vi "Main Page.vi"(8 "error in (no error)":errorcluster, 11 "Node Ptr":T3 format="%.0x") -> (0 "error out":errorcluster)   [LabVIEW 2018, in "Instrument Addon System Explorer.lvlib"]
uses:
  Instrument Addon System Explorer.lvlib
  <vilib>/NI Veristand/Custom Device API/Custom Device Item Ref.ctl
  Addon Shared/Types/FG Control.ctl
  <vilib>/NI/NI VeriStand Hardware Resource Discovery/_Types/Filter Type.ctl
  Addon Shared/SubVIs/Constants.vi
  <vilib>/NI/NI VeriStand Advanced SysDef API/SysDef API/SysDef.Property.Get.vi
  <vilib>/NI/NI VeriStand Advanced SysDef API/_SubVIs/SysDef.Property.Get.String.vi
  <vilib>/NI/NI VeriStand Advanced SysDef API/SysDef API/SysDef.Property.Set.vi
  <vilib>/NI/NI VeriStand Advanced SysDef API/_SubVIs/SysDef.Property.Set.String.vi
  <vilib>/NI Veristand/Custom Device API/NI VeriStand - Get Item Property.vi
  <vilib>/NI Veristand/Custom Device API/Get Item Property (Boolean).vi
  <vilib>/NI Veristand/Custom Device API/Get Item Property (U32).vi
  <vilib>/NI Veristand/Custom Device API/Get Item Property (String).vi
  <vilib>/NI Veristand/Custom Device API/NI VeriStand - Set Item Property.vi
  <vilib>/NI Veristand/Custom Device API/Set Item Property (Boolean).vi
  <vilib>/NI Veristand/Custom Device API/Set Item Property (U32).vi
  <vilib>/NI Veristand/Custom Device API/Set Item Property (String).vi
  <vilib>/Utility/LVClass/Get LV Class Default Value.vi
  Support Libraries/Protocols.lvlibp/Protocol Parent/Protocol Parent.lvclass
  <vilib>/NI Veristand/Custom Device API/Custom Device API.lvlib
  Addon Shared/Instrument Addon Shared.lvlib
  <vilib>/NI/NI VeriStand Hardware Resource Discovery/NIVS Hardware Discovery.lvlib
  APIs/Scripting API/Instrument Addon Scripting API.lvlib
panel:
  out "Version":string
  in  "PCL Decimation":u32=1 min=1 max=10000 step=1
  in  "Protocol Settings":T1(tab)=enum."TCP/IP"
  in  "COM Browse":bool
  in  "Termination Character":u8=10 format="%.0x"
  in  "End Write":bool=TRUE caption="End Write on Termination Character?"
  in  "End Read":bool=TRUE caption="End Read on Termination Character?"
  in  "XOFF":T2(ring)=enum."DC3"
  in  "XON":T2(ring)=enum."DC1"
  in  "Flow Control":u16(ring) items=["None"=0, "XON/XOFF"=1, "RTS/CTS"=2, "DTR/DSR"=4]
  in  "Stop Bits":u16(ring)=10 items=["1.0"=10, "1.5"=15, "2.0"=20]
  in  "Parity":enum16{"None", "Odd", "Even", "Mark", "Space"}(ring)
  in  "Data Bits":u16=8 min=5 max=8 step=1
  in  "Baud Rate":u32(ring)=9600 items=["75"=75, "110"=110, "134"=134, "150"=150, "300"=300, "600"=600, "1200"=1200, "1800"=1800, "2400"=2400, "4800"=4800, "7200"=7200, "9600"=9600, "14400"=14400, "19200"=19200, "28800"=28800, "38400"=38400, "56000"=56000, "57600"=57600, "115200"=115200, "128000"=128000, "230400"=230400, "460800"=460800, "921600"=921600, "1843200"=1843200, "3000000"=3000000]
  in  "Port":string="COM1"
  in  "VISA Browse":bool
  in  "Append Write Termination Character":bool caption="Append Write Termination Character?"
  in  "Timeout":u32=2000 caption="Timeout (ms)"
  in  "Termination Character":u8=10 format="%.0x"
  in  "Enable Termination Character":bool=TRUE caption="Enable Termination Character?"
  in  "VISA Resource":string="GPIB0::2::INSTR"
  in  "Port":u16
  in  "IP Address":string="localhost"
  in  "UDP Browse":bool
  in  "Target Port":u16
  in  "Target IP Address":string="localhost"
  in  "Local Port":u16
  in  "Local IP Address":string="localhost"
  in  "Assert REN w/ IFC":bool=TRUE caption="Assert REN w/ IFC?"
  in  "IST Bit Sense":bool=TRUE caption="IST Bit Sense?"
  in  "System Controller":bool=TRUE caption="System Controller?"
  in  "GPIB Address":string="1"
  in  "ConvBox Address":string="0"
  in  "ConvBox Browse":bool
  in  "ConvBox Port":string="COM1"
  in  "Protocol":string(combo)
  in  "SHDocVw.IWebBrowser":refnum<k7>(container)
  in  "Header":cluster{"Section Name":string}={"Section Name"="Addon Settings"}
  in  "Description":string
  in  "Name":string
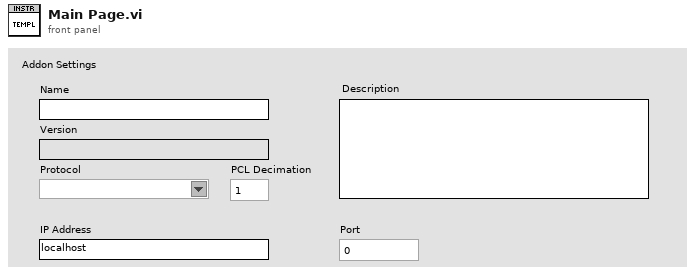
[diagram p1: front panel]
types:
  T1 = enum32{"RS232", "VISA", "TCP/IP", "UDP", "ConvBox"}
  T2 = enum16{"NUL", "SOH", "STX", "ETX", "EOT", "ENQ", "ACK", "BEL", "BS", "HT", "LF", "VT", "FF", "CR", "SO", "SI", "DLE", "DC1", "DC2", "DC3", "DC4", "NAK", "SYN", "ETB", "CAN", "EM", "SUB", "ESC", "FS", "GS", "RS", "US", "SP", "!", "\"", "#", "$", "%", "&", "'", "(", ")", "*", "+", ",", "- (-)", ".", "/", "0", "1", "2", "3", "4", "5", "6", "7", "8", "9", ":", ";", "<", "=", ">", "?", "@", "A", "B", "C", "D", "E", "F", "G", "H", "I", "J", "K", "L", "M", "N", "O", "P", "Q", "R", "S", "T", "U", "V", "W", "X", "Y", "Z", "[", "\\", "]", "^", "_", "`", "a", "b", "c", "d", "e", "f", "g", "h", "i", "j", "k", "l", "m", "n", "o", "p", "q", "r", "s", "t", "u", "v", "w", "x", "y", "z", "{", "|", "}", "~"}
  T3 = typedef "Custom Device API.lvlib/Custom Device Item Ref.ctl" = u64
  T4 = typedef "Custom Device API.lvlib/Custom Device Item Info.ctl" = cluster{"Name":string, "Is Channel":bool, "GUID":string, "Is Waveform":bool}
  T5 = typedef "Instrument Addon Shared.lvlib/FG Control.ctl" = enum16{"Get", "Set"}
  T6 = typedef "NIVS Hardware Discovery.lvlib/Filter Type.ctl" = enum16{"Device Category", "Product Name", "Ethernet", "XNET", "VISA", "FPGA", "EtherCAT Master", "DAQmx", "GPIB", "Serial"}
  T7 = typedef "Custom Device API.lvlib/Custom Device Commands.ctl" = enum16{"Default", "Item renamed", "Shutdown", "Dynamic button pressed"}
  T8 = typedef "Instrument Addon Shared.lvlib/VISA Settings.ctl" = cluster{"VISA Resource":string, "Enable Termination Character":bool, "Termination Character":u8, "Timeout":u32, "Append Write Termination Character":bool}
  T9 = typedef "Instrument Addon Shared.lvlib/TCPIP Settings.ctl" = cluster{"IP Address":string, "Port":u16}
  T10 = typedef "Instrument Addon Shared.lvlib/UDP Settings.ctl" = cluster{"Local IP Address":string, "Local Port":u16, "Target IP Address":string, "Target Port":u16}
  T11 = typedef "Instrument Addon Shared.lvlib/RSXXX Port Settings.ctl" = cluster{"Port":string, "Baud Rate":u32, "Data Bits":u16, "Parity":enum16{"None", "Odd", "Even", "Mark", "Space"}, "Stop Bits":u16, "Flow Control":u16, "XON":enum16{"NUL", "SOH", "STX", "ETX", "EOT", "ENQ", "ACK", "BEL", "BS", "HT", "LF", "VT", "FF", "CR", "SO", "SI", "DLE", "DC1", "DC2", "DC3", "DC4", "NAK", "SYN", "ETB", "CAN", "EM", "SUB", "ESC", "FS", "GS", "RS", "US", "SP", "!", "\"", "#", "$", "%", "&", "'", "(", ")", "*", "+", ",", "- (-)", ".", "/", "0", "1", "2", "3", "4", "5", "6", "7", "8", "9", ":", ";", "<", "=", ">", "?", "@", "A", "B", "C", "D", "E", "F", "G", "H", "I", "J", "K", "L", "M", "N", "O", "P", "Q", "R", "S", "T", "U", "V", "W", "X", "Y", "Z", "[", "\\", "]", "^", "_", "`", "a", "b", "c", "d", "e", "f", "g", "h", "i", "j", "k", "l", "m", "n", "o", "p", "q", "r", "s", "t", "u", "v", "w", "x", "y", "z", "{", "|", "}", "~"}, "XOFF":enum16{"NUL", "SOH", "STX", "ETX", "EOT", "ENQ", "ACK", "BEL", "BS", "HT", "LF", "VT", "FF", "CR", "SO", "SI", "DLE", "DC1", "DC2", "DC3", "DC4", "NAK", "SYN", "ETB", "CAN", "EM", "SUB", "ESC", "FS", "GS", "RS", "US", "SP", "!", "\"", "#", "$", "%", "&", "'", "(", ")", "*", "+", ",", "- (-)", ".", "/", "0", "1", "2", "3", "4", "5", "6", "7", "8", "9", ":", ";", "<", "=", ">", "?", "@", "A", "B", "C", "D", "E", "F", "G", "H", "I", "J", "K", "L", "M", "N", "O", "P", "Q", "R", "S", "T", "U", "V", "W", "X", "Y", "Z", "[", "\\", "]", "^", "_", "`", "a", "b", "c", "d", "e", "f", "g", "h", "i", "j", "k", "l", "m", "n", "o", "p", "q", "r", "s", "t", "u", "v", "w", "x", "y", "z", "{", "|", "}", "~"}, "End Read on Termination Character":bool, "End Write on Termination Character":bool, "Termination Character":u8}
  T12 = typedef "Instrument Addon Shared.lvlib/GPIB ConvBox Settings.ctl" = cluster{"Port":string, "ConvBox Address":string, "Assert Ren with IFC":bool, "System controller":bool, "IST bit sense":bool, "GPIB Address":string}
  T13 = typedef "Protocols.lvlibp/Protocol Parent.lvclass/Base Protocol Type.ctl" = enum16{"RS-XXX", "VISA", "TCPIP", "UDP", "GPIB ConvBox"}
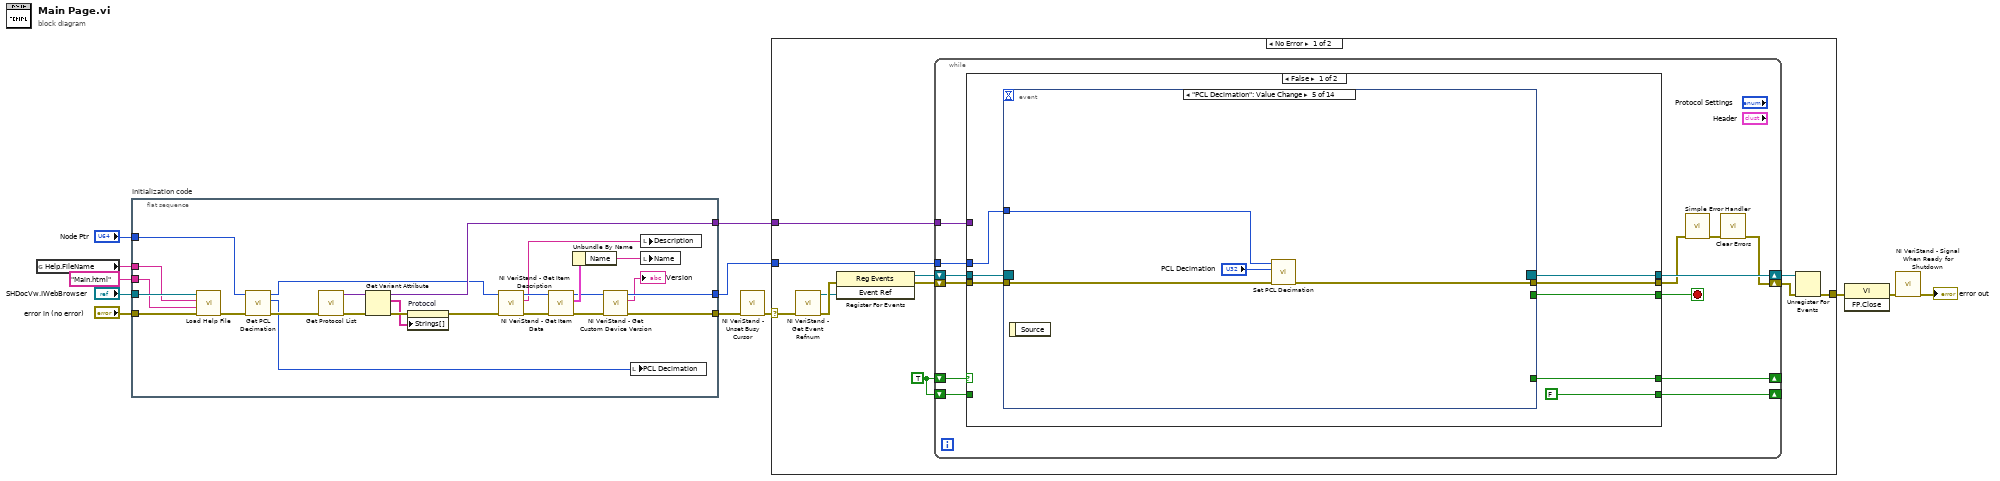
[diagram p0: block diagram]
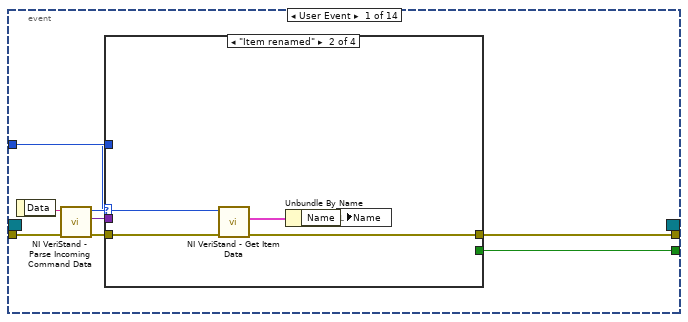
[diagram p2: hidden frame]
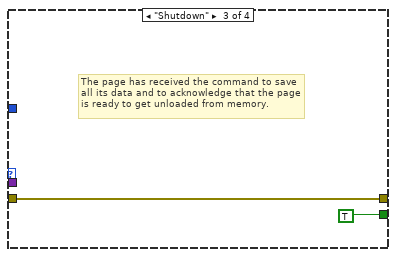
[diagram p4: hidden frame]
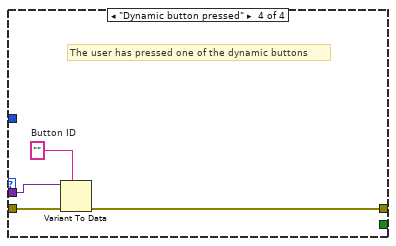
[diagram p5: hidden frame]
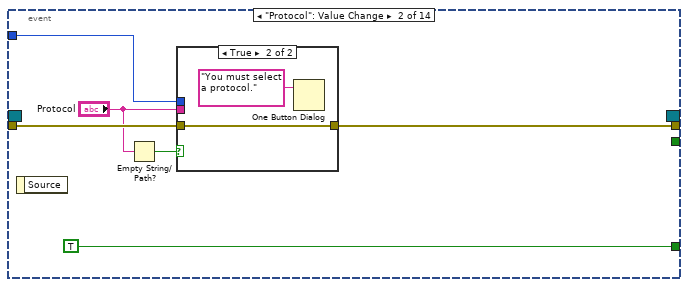
[diagram p6: hidden frame]
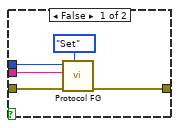
[diagram p7: hidden frame]
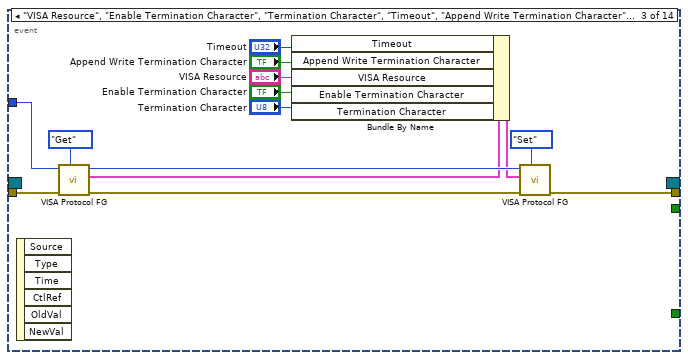
[diagram p8: hidden frame]
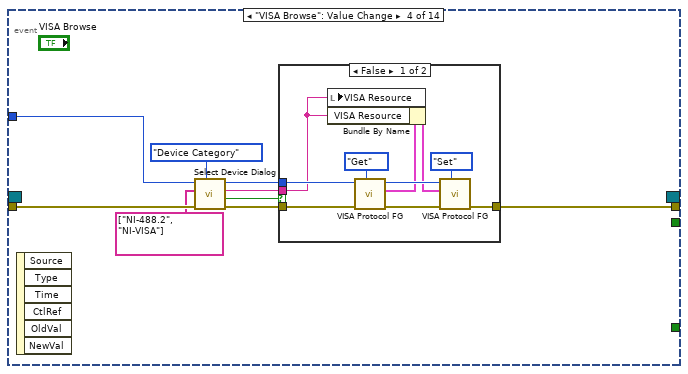
[diagram p9: hidden frame]
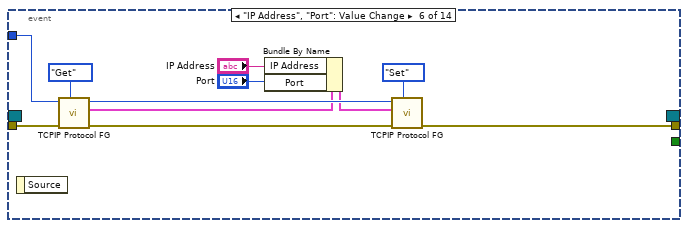
[diagram p11: hidden frame]
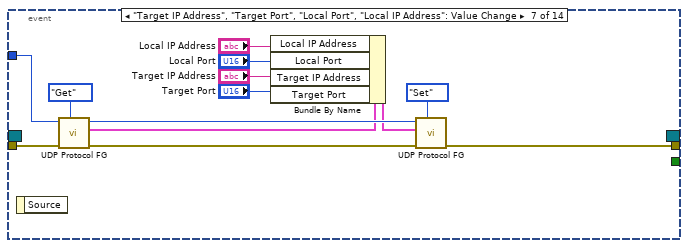
[diagram p12: hidden frame]
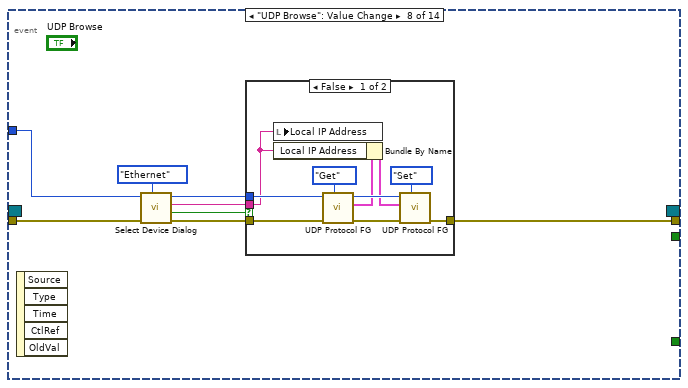
[diagram p13: hidden frame]
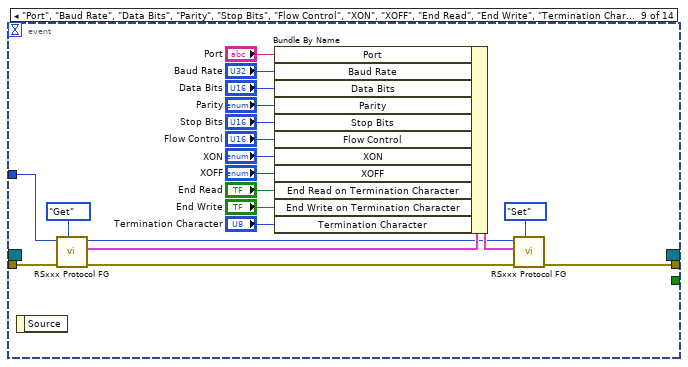
[diagram p15: hidden frame]
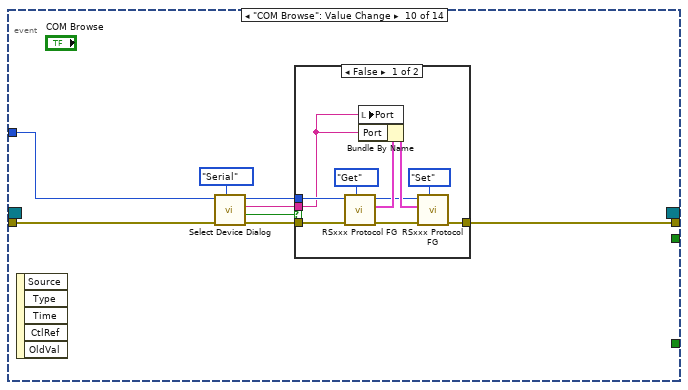
[diagram p16: hidden frame]
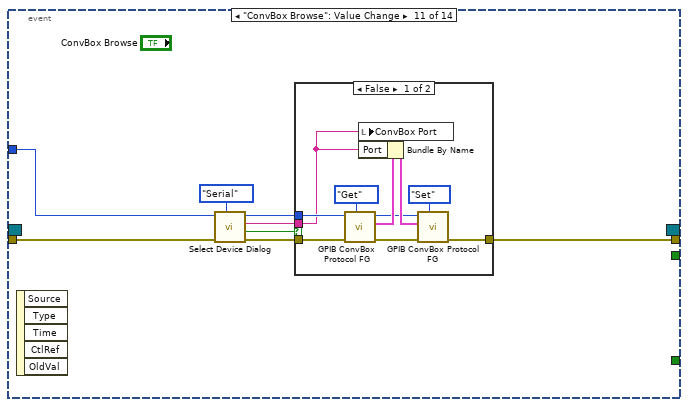
[diagram p18: hidden frame]
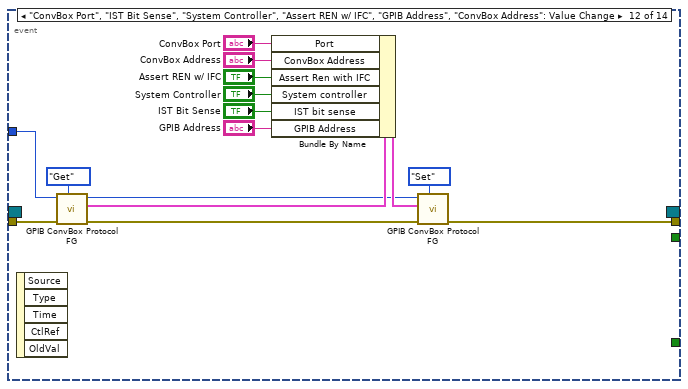
[diagram p20: hidden frame]
diagram:
  n1 = global read "Constants.vi" "Help.FileName"() -> (w1:string)
  n2 = flat-sequence "Initialization code" {
    tunnel: "error in (no error)" -> [w32]
    tunnel: "Node Ptr" -> [w16]
    tunnel: [w21] -> w8
    tunnel: [w19] -> w5
    tunnel: "SHDocVw.IWebBrowser" -> [w31]
    tunnel: "Main.html" ("HTML File") -> [w30]
    tunnel: w1 -> [w29]
    tunnel: [w24] -> w2
    frame #0 {
      n3 = call "Load Help File.vi"("error in (no error)"=w32, "HTML File"=w30, "Main CHM File"=w29, "SHDocVw.IWebBrowser2"=w31) -> ("error out"=w15:errorcluster)  [unwired: 7 in]
      n4 = call "Get PCL Decimation.vi"("Error In"=w15, "Instrument Addon Refnum In"=w16) -> ("Error Out"=w14:errorcluster, "PCL Decimation"=w13:u32, "Instrument Addon Refnum Out"=w17:T3)  [unwired: 7 in]
      n5 = call "Get Protocol List.vi"("error in (no error)"=w14) -> ("error out"=w27:errorcluster, "Class Lookup"=w28:variant)  [unwired: 9 in]
      n6 = Get Variant Attribute(Variant=w28, error in=w27) -> (duplicate Variant=w24:variant, names=w25:string[], error out=w26:errorcluster)  [unwired: 2 in, 1 out]
      n7 = property on="Protocol" class="CmbBox"(error in=w26, "Strings[]"=w25) -> (error out=w23:errorcluster)  [unwired: 1 in, 1 out]
      n8 = call <vilib>:"NI VeriStand - Get Item Description.vi"("error in (no error)"=w23, "Item Ref in"=w17) -> ("error out"=w35:errorcluster, "Description"=w36:string, "Item Ref out"=w37:T3)  [unwired: 7 out]
      n9 = call <vilib>:"NI VeriStand - Get Item Data.vi"("error in (no error)"=w35, "Item Ref in"=w37) -> ("error out"=w22:errorcluster, "Item Info"=w34:T4, "Item Ref out"=w20:T3)  [unwired: 7 out]
      n10 = Unbundle By Name(w34) -> ("Name"=w33:string)
      n11 = call <vilib>:"NI VeriStand - Get Custom Device Version.vi"("error in (no error)"=w22, "Device Ref in"=w20) -> ("error out"=w21:errorcluster, "Value"=→"Version":string, "Device Ref out"=w19:T3)  [unwired: 7 in]
      n12 = local write "PCL Decimation"(w13) -> ()
      n13 = local write "Description"(w36) -> ()
      n14 = local write "Name"(w33) -> ()
    }
  }
  n15 = call <vilib>:"NI VeriStand - Unset Busy Cursor.vi"("error in (no error)"=w8) -> ("error out"=w7:errorcluster)  [unwired: 10 out]
  n16 = case shown="No Error" w7 {
    selector: w7 -> [w40 w347]
    tunnel: [w45 w345] -> w12
    tunnel: w5 -> [w41 _]
    tunnel: w2 -> [w39 _]
    frame No Error {
      w38 = TRUE
      n17 = call <vilib>:"NI VeriStand - Get Event Refnum.vi"("error in (no error)"=w40) -> ("error out"=w48:errorcluster, "Event Ref"=w44:refnum<user-event>)  [unwired: 9 out]
      n18 = register-events(error in=w48, w44) -> (reference out=w42:refnum<event-registration>, error out=w43:errorcluster)  [unwired: 1 in]
      n19 = while {
        tunnel: w41 -> [w57]
        shift-right: [w54] -> w46
        shift-left: w43 -> [w60]
        shift-right: [w61] -> w47
        shift-left: w42 -> [w59]
        tunnel: w39 -> [w53]
        shift-right: [w51] -> _
        shift-left: w38 -> [w52]
        shift-right: [w49] -> _
        shift-left: w38 -> [w50]
        stop <- w58 stop-if-true
        n20 = case shown="False" w52 {
          tunnel: [w69 w272] -> w61
          tunnel: w60 -> [w68 w280]
          tunnel: w59 -> [w67 w272]
          tunnel: [w66 _] -> w58
          tunnel: w57 -> [w65 w279]
          tunnel: [w64 w267] -> w56
          tunnel: w53 -> [_ w277]
          tunnel: [w63 w265] -> w51
          tunnel: w50 -> [_ w266]
          tunnel: [FALSE w265] -> w49
          frame False {
            n21 = event shown="[4] \"PCL Decimation\": Value Change" {
              selector: w67 -> [_ _ _ _ _ _ _ _ _ _ _ _ _ _]
              dyn-events: [_ _ _ _ _ _ _ _ _ _ _ _ _ _] -> w69
              timeout: _ -> [_ _ _ _ _ _ _ _ _ _ _ _ _ _]
              tunnel: w68 -> [w77 w94 w115 w124 w139 w150 w163 w171 w200 w210 w229 w249 w260 w263]
              tunnel: [w73 _ _ _ _ _ _ _ _ _ _ _ _ _] -> w66
              tunnel: [w72 w90 w111 w125 w138 w146 w159 w172 w202 w211 w230 w256 w259 w262] -> w64
              tunnel: w65 -> [w71 w95 w114 w122 w137 w149 w162 w169 w198 w209 w228 w248 w258 w264]
              tunnel: [_ TRUE _ _ _ _ _ _ _ _ _ _ _ _] -> w63
              event User Event {
                n22 = event-data() -> ("Data"=w76:string)  [unwired: 1 out]
                n23 = call <vilib>:"NI VeriStand - Parse Incoming Command Data.vi"("error in (no error)"=w77, "Incoming data"=w76) -> ("error out"=w75:errorcluster, "Outgoing data"=w70:variant, "Action"=w74:T7)  [unwired: 7 out]
                n24 = case shown="\"Item renamed\"" w74 {
                  tunnel: w75 -> [w78 w83 w84 w89]
                  tunnel: [_ _ TRUE _] -> w73
                  tunnel: [w78 w80 w84 w86] -> w72
                  tunnel: w71 -> [_ w82 _ _]
                  tunnel: w70 -> [_ _ _ w88]
                  frame "Default", Default {
                  }
                  frame "Item renamed" {
                    n25 = call <vilib>:"NI VeriStand - Get Item Data.vi"("error in (no error)"=w83, "Item Ref in"=w82) -> ("error out"=w80:errorcluster, "Item Info"=w81:T4)  [unwired: 8 out]
                    n26 = Unbundle By Name(w81) -> ("Name"=w79:string)
                    n27 = local write "Name"(w79) -> ()
                  }
                  frame "Shutdown" {
                    # "The page has received the command to save all its data and to acknowledge that the page is ready to get unloaded from memory."
                  }
                  frame "Dynamic button pressed" {
                    w87 = ""  # Button ID
                    # "The user has pressed one of the dynamic buttons"
                    n28 = Variant To Data(error in=w89, type=w87, Variant=w88) -> (error out=w86:errorcluster)  [unwired: 1 out]
                  }
                }
              }
              event "Protocol": Value Change {
                n29 = event-data() -> ()  [unwired: 2 out]
                n30 = Empty String/Path?(string/path="Protocol") -> (empty?=w92:bool)
                n31 = case shown="True" w92 {
                  tunnel: w95 -> [w98 _]
                  tunnel: w94 -> [w99 w101]
                  tunnel: [w96 w101] -> w90
                  tunnel: "Protocol" -> [w97 _]
                  frame False {
                    n32 = call "Protocol FG.vi"("Action"=FG_Control."Set", "error in (no error)"=w99, "Protocol"=w97, "Device Item Ref in"=w98) -> ("error out"=w96:errorcluster)  [unwired: 5 in, 2 out]
                  }
                  frame True {
                    n33 = One Button Dialog(message="You must select a protocol.") -> ()  [unwired: 1 in, 1 out]
                  }
                }
              }
              event "VISA Resource", "Enable Termination Character", "Termination Character", "Timeout", "Append Write Termination Character": Value Change {
                n34 = event-data() -> ()  [unwired: 7 out]
                n35 = call "VISA Protocol FG.vi"("Action"=FG_Control."Get", "error in (no error)"=w115, "Device Item Ref in"=w114) -> ("error out"=w112:errorcluster, "VISA Config"=w109:T8, "Item Ref out"=w110:T3)  [unwired: 6 in]
                n36 = Bundle By Name(cluster=w109, "Timeout"="Timeout", "Append Write Termination Character"="Append Write Termination Character", "VISA Resource"="VISA Resource", "Enable Termination Character"="Enable Termination Character", "Termination Character"="Termination Character") -> (w108:T8)
                n37 = call "VISA Protocol FG.vi"("Action"=FG_Control."Set", "error in (no error)"=w112, "VISA Config"=w108, "Device Item Ref in"=w110) -> ("error out"=w111:errorcluster)  [unwired: 5 in, 2 out]
              }
              event "VISA Browse": Value Change {
                n38 = event-data() -> ()  [unwired: 7 out]
                n39 = call <vilib>:"Select Device Dialog.vi"("Filter Type"=Filter_Type."Device Category", "error in (no error)"=w124, "Filter Names"=string[] ["NI-488.2", "NI-VISA"], "Item Ref in"=w122) -> ("error out"=w123:errorcluster, "Cancelled?"=w120:bool, "Selected Alias"=w119:string, "Item Ref out"=w121:T3)  [unwired: 4 in]
                n40 = case shown="False" w120 {
                  tunnel: w123 -> [w134 w136]
                  tunnel: w121 -> [w133 _]
                  tunnel: [w130 w136] -> w125
                  tunnel: w119 -> [w126 _]
                  frame False {
                    n41 = local write "VISA Resource"(w126) -> ()
                    n42 = call "VISA Protocol FG.vi"("Action"=FG_Control."Get", "error in (no error)"=w134, "Device Item Ref in"=w133) -> ("error out"=w131:errorcluster, "VISA Config"=w128:T8, "Item Ref out"=w129:T3)  [unwired: 6 in]
                    n43 = Bundle By Name(cluster=w128, "VISA Resource"=w126) -> (w127:T8)
                    n44 = call "VISA Protocol FG.vi"("Action"=FG_Control."Set", "error in (no error)"=w131, "VISA Config"=w127, "Device Item Ref in"=w129) -> ("error out"=w130:errorcluster)  [unwired: 5 in, 2 out]
                  }
                  frame True {
                  }
                }
              }
              event "PCL Decimation": Value Change {
                n45 = event-data() -> ()  [unwired: 2 out]
                n46 = call "Set PCL Decimation.vi"("Error In"=w139, "PCL Decimation"="PCL Decimation", "Instrument Addon Refnum In"=w137) -> ("Error Out"=w138:errorcluster)  [unwired: 7 in, 1 out]
              }
              event "IP Address", "Port": Value Change {
                n47 = event-data() -> ()  [unwired: 2 out]
                n48 = call "TCPIP Protocol FG.vi"("Action"=FG_Control."Get", "error in (no error)"=w150, "Device Item Ref in"=w149) -> ("error out"=w147:errorcluster, "TCP/IP Config"=w144:T9, "Item Ref out"=w145:T3)  [unwired: 6 in]
                n49 = Bundle By Name(cluster=w144, "IP Address"="IP Address", "Port"="Port") -> (w143:T9)
                n50 = call "TCPIP Protocol FG.vi"("Action"=FG_Control."Set", "error in (no error)"=w147, "TCP/IP Config"=w143, "Device Item Ref in"=w145) -> ("error out"=w146:errorcluster)  [unwired: 5 in, 2 out]
              }
              event "Target IP Address", "Target Port", "Local Port", "Local IP Address": Value Change {
                n51 = event-data() -> ()  [unwired: 2 out]
                n52 = call "UDP Protocol FG.vi"("Action"=FG_Control."Get", "error in (no error)"=w163, "Device Item Ref in"=w162) -> ("error out"=w160:errorcluster, "UDP Config"=w157:T10, "Item Ref out"=w158:T3)  [unwired: 6 in]
                n53 = Bundle By Name(cluster=w157, "Local IP Address"="Local IP Address", "Local Port"="Local Port", "Target IP Address"="Target IP Address", "Target Port"="Target Port") -> (w156:T10)
                n54 = call "UDP Protocol FG.vi"("Action"=FG_Control."Set", "error in (no error)"=w160, "UDP Config"=w156, "Device Item Ref in"=w158) -> ("error out"=w159:errorcluster)  [unwired: 5 in, 2 out]
              }
              event "UDP Browse": Value Change {
                n55 = event-data() -> ()  [unwired: 6 out]
                n56 = call <vilib>:"Select Device Dialog.vi"("Filter Type"=Filter_Type."Ethernet", "error in (no error)"=w171, "Item Ref in"=w169) -> ("error out"=w170:errorcluster, "Cancelled?"=w167:bool, "Selected Alias"=w166:string, "Item Ref out"=w168:T3)  [unwired: 5 in]
                n57 = case shown="False" w167 {
                  tunnel: w170 -> [w181 w183]
                  tunnel: w168 -> [w180 _]
                  tunnel: [w177 w183] -> w172
                  tunnel: w166 -> [w173 _]
                  frame False {
                    n58 = local write "Local IP Address"(w173) -> ()
                    n59 = call "UDP Protocol FG.vi"("Action"=FG_Control."Get", "error in (no error)"=w181, "Device Item Ref in"=w180) -> ("error out"=w178:errorcluster, "UDP Config"=w175:T10, "Item Ref out"=w176:T3)  [unwired: 6 in]
                    n60 = Bundle By Name(cluster=w175, "Local IP Address"=w173) -> (w174:T10)
                    n61 = call "UDP Protocol FG.vi"("Action"=FG_Control."Set", "error in (no error)"=w178, "UDP Config"=w174, "Device Item Ref in"=w176) -> ("error out"=w177:errorcluster)  [unwired: 5 in, 2 out]
                  }
                  frame True {
                  }
                }
              }
              event "Port", "Baud Rate", "Data Bits", "Parity", "Stop Bits", "Flow Control", "XON", "XOFF", "End Read", "End Write", "Termination Character": Value Change {
                n62 = event-data() -> ()  [unwired: 2 out]
                n63 = call "RSxxx Protocol FG.vi"("Action"=FG_Control."Get", "error in (no error)"=w200, "Device Item Ref in"=w198) -> ("error out"=w199:errorcluster, "Serial Config"=w197:T11, "Item Ref out"=w184:T3)  [unwired: 6 in]
                n64 = Bundle By Name(cluster=w197, "Port"="Port", "Baud Rate"="Baud Rate", "Data Bits"="Data Bits", "Parity"="Parity", "Stop Bits"="Stop Bits", "Flow Control"="Flow Control", "XON"="XON", "XOFF"="XOFF", "End Read on Termination Character"="End Read", "End Write on Termination Character"="End Write", "Termination Character"="Termination Character") -> (w196:T11)
                n65 = call "RSxxx Protocol FG.vi"("Action"=FG_Control."Set", "error in (no error)"=w199, "Serial Config"=w196, "Device Item Ref in"=w184) -> ("error out"=w202:errorcluster)  [unwired: 5 in, 2 out]
              }
              event "COM Browse": Value Change {
                n66 = event-data() -> ()  [unwired: 6 out]
                n67 = call <vilib>:"Select Device Dialog.vi"("Filter Type"=Filter_Type."Serial", "error in (no error)"=w210, "Item Ref in"=w209) -> ("error out"=w207:errorcluster, "Cancelled?"=w206:bool, "Selected Alias"=w205:string, "Item Ref out"=w208:T3)  [unwired: 5 in]
                n68 = case shown="False" w206 {
                  tunnel: [w220 w222] -> w211
                  tunnel: w207 -> [w218 w222]
                  tunnel: w208 -> [w216 _]
                  tunnel: w205 -> [w212 _]
                  frame False {
                    n69 = call "RSxxx Protocol FG.vi"("Action"=FG_Control."Get", "error in (no error)"=w218, "Device Item Ref in"=w216) -> ("error out"=w217:errorcluster, "Serial Config"=w215:T11, "Item Ref out"=w213:T3)  [unwired: 6 in]
                    n70 = local write "Port"(w212) -> ()
                    n71 = Bundle By Name(cluster=w215, "Port"=w212) -> (w214:T11)
                    n72 = call "RSxxx Protocol FG.vi"("Action"=FG_Control."Set", "error in (no error)"=w217, "Serial Config"=w214, "Device Item Ref in"=w213) -> ("error out"=w220:errorcluster)  [unwired: 5 in, 2 out]
                  }
                  frame True {
                  }
                }
              }
              event "ConvBox Browse": Value Change {
                n73 = event-data() -> ()  [unwired: 6 out]
                n74 = call <vilib>:"Select Device Dialog.vi"("Filter Type"=Filter_Type."Serial", "error in (no error)"=w229, "Item Ref in"=w228) -> ("error out"=w226:errorcluster, "Cancelled?"=w225:bool, "Selected Alias"=w224:string, "Item Ref out"=w227:T3)  [unwired: 5 in]
                n75 = case shown="False" w225 {
                  tunnel: [w239 w241] -> w230
                  tunnel: w226 -> [w237 w241]
                  tunnel: w227 -> [w235 _]
                  tunnel: w224 -> [w231 _]
                  frame False {
                    n76 = call "GPIB ConvBox Protocol FG.vi"("Action"=FG_Control."Get", "error in (no error)"=w237, "Device Item Ref in"=w235) -> ("error out"=w236:errorcluster, "GPIB ConvBox Config"=w234:T12, "Item Ref out"=w232:T3)  [unwired: 6 in]
                    n77 = local write "ConvBox Port"(w231) -> ()
                    n78 = Bundle By Name(cluster=w234, "Port"=w231) -> (w233:T12)
                    n79 = call "GPIB ConvBox Protocol FG.vi"("Action"=FG_Control."Set", "error in (no error)"=w236, "GPIB ConvBox Config"=w233, "Device Item Ref in"=w232) -> ("error out"=w239:errorcluster)  [unwired: 5 in, 2 out]
                  }
                  frame True {
                  }
                }
              }
              event "ConvBox Port", "IST Bit Sense", "System Controller", "Assert REN w/ IFC", "GPIB Address", "ConvBox Address": Value Change {
                n80 = event-data() -> ()  [unwired: 6 out]
                n81 = call "GPIB ConvBox Protocol FG.vi"("Action"=FG_Control."Get", "error in (no error)"=w249, "Device Item Ref in"=w248) -> ("error out"=w253:errorcluster, "GPIB ConvBox Config"=w252:T12, "Item Ref out"=w250:T3)  [unwired: 6 in]
                n82 = Bundle By Name(cluster=w252, "Port"="ConvBox Port", "ConvBox Address"="ConvBox Address", "Assert Ren with IFC"="Assert REN w/ IFC", "System controller"="System Controller", "IST bit sense"="IST Bit Sense", "GPIB Address"="GPIB Address") -> (w251:T12)
                n83 = call "GPIB ConvBox Protocol FG.vi"("Action"=FG_Control."Set", "error in (no error)"=w253, "GPIB ConvBox Config"=w251, "Device Item Ref in"=w250) -> ("error out"=w256:errorcluster)  [unwired: 5 in, 2 out]
              }
              event "Name": Value Change {
                n84 = event-data() -> ()  [unwired: 2 out]
                n85 = call <vilib>:"NI VeriStand - Rename Custom Device Item.vi"("error in (no error)"=w260, "New Name"="Name", "Item Ref in"=w258) -> ("error out"=w259:errorcluster)  [unwired: 1 in, 7 out]
              }
              event "Description": Value Change {
                n86 = event-data() -> ()  [unwired: 2 out]
                n87 = call <vilib>:"NI VeriStand - Set Item Description.vi"("error in (no error)"=w263, "Description"="Description", "Item Ref in"=w264) -> ("error out"=w262:errorcluster)  [unwired: 8 out]
              }
            }
          }
          frame True {
            w265 = FALSE
            n88 = call "Protocol FG.vi"("Action"=FG_Control."Get", "error in (no error)"=w280, "Device Item Ref in"=w279) -> ("error out"=w276:errorcluster, "Protocol out"=w273:string, "Item Ref out"=w275:T3)  [unwired: 6 in]
            n89 = call "Lookup Base Protocol Class and Info.vi"("error in (no error)"=w276, "Protocol in"=w273, "Class Lookup"=w277) -> ("error out"=w278:errorcluster, "Protocol out"=w271:T13, "Error Codes"=w270:cluster{"Code":i32, "String":string}[])  [unwired: 4 in, 2 out]
            n90 = case shown="\"VISA\"" w271 {
              tunnel: w278 -> [w297 w305 w315 w332 w344]
              tunnel: [w296 w304 w314 w331 w343] -> w268
              tunnel: w275 -> [w295 w303 w313 w330 w342]
              tunnel: [w287 w298 w306 w316 w333] -> w269
              frame "VISA" {
                n91 = call "VISA Protocol FG.vi"("Action"=FG_Control."Get", "error in (no error)"=w297, "Device Item Ref in"=w295) -> ("error out"=w296:errorcluster, "VISA Config"=w293:T8, "Item Ref out"=w287:T3)  [unwired: 6 in]
                n92 = Unbundle By Name(w293) -> ("Append Write Termination Character"=w288:bool, "Timeout"=w289:u32, "VISA Resource"=w292:string, "Enable Termination Character"=w291:bool, "Termination Character"=w290:u8)
                n93 = local write "Append Write Termination Character"(w288) -> ()
                n94 = local write "Enable Termination Character"(w291) -> ()
                n95 = local write "Termination Character"(w290) -> ()
                n96 = local write "Timeout"(w289) -> ()
                n97 = local write "VISA Resource"(w292) -> ()
              }
              frame "TCPIP" {
                n98 = call "TCPIP Protocol FG.vi"("Action"=FG_Control."Get", "error in (no error)"=w305, "Device Item Ref in"=w303) -> ("error out"=w304:errorcluster, "TCP/IP Config"=w301:T9, "Item Ref out"=w298:T3)  [unwired: 6 in]
                n99 = Unbundle By Name(w301) -> ("IP Address"=w300:string, "Port"=w299:u16)
                n100 = local write "IP Address"(w300) -> ()
                n101 = local write "Port"(w299) -> ()
              }
              frame "UDP" {
                n102 = call "UDP Protocol FG.vi"("Action"=FG_Control."Get", "error in (no error)"=w315, "Device Item Ref in"=w313) -> ("error out"=w314:errorcluster, "UDP Config"=w311:T10, "Item Ref out"=w306:T3)  [unwired: 6 in]
                n103 = Unbundle By Name(w311) -> ("Local IP Address"=w310:string, "Local Port"=w309:u16, "Target IP Address"=w308:string, "Target Port"=w307:u16)
                n104 = local write "Local IP Address"(w310) -> ()
                n105 = local write "Local Port"(w309) -> ()
                n106 = local write "Target IP Address"(w308) -> ()
                n107 = local write "Target Port"(w307) -> ()
              }
              frame "RS-XXX" {
                n108 = call "RSxxx Protocol FG.vi"("Action"=FG_Control."Get", "error in (no error)"=w332, "Device Item Ref in"=w330) -> ("error out"=w331:errorcluster, "Serial Config"=w328:T11, "Item Ref out"=w316:T3)  [unwired: 6 in]
                n109 = Unbundle By Name(w328) -> ("Port"=w327:string, "Baud Rate"=w326:u32, "Data Bits"=w317:u16, "Parity"=w318:enum16{"None", "Odd", "Even", "Mark", "Space"}, "Stop Bits"=w319:u16, "Flow Control"=w320:u16, "XON"=w321:T2, "XOFF"=w322:T2, "End Read on Termination Character"=w323:bool, "End Write on Termination Character"=w324:bool, "Termination Character"=w325:u8)
                n110 = local write "Termination Character"(w325) -> ()
                n111 = local write "Flow Control"(w320) -> ()
                n112 = local write "Data Bits"(w317) -> ()
                n113 = local write "Stop Bits"(w319) -> ()
                n114 = local write "XON"(w321) -> ()
                n115 = local write "End Write"(w324) -> ()
                n116 = local write "Port"(w327) -> ()
                n117 = local write "Baud Rate"(w326) -> ()
                n118 = local write "Parity"(w318) -> ()
                n119 = local write "XOFF"(w322) -> ()
                n120 = local write "End Read"(w323) -> ()
              }
              frame "GPIB ConvBox" {
                n121 = call "GPIB ConvBox Protocol FG.vi"("Action"=FG_Control."Get", "error in (no error)"=w344, "Device Item Ref in"=w342) -> ("error out"=w343:errorcluster, "GPIB ConvBox Config"=w340:T12, "Item Ref out"=w333:T3)  [unwired: 6 in]
                n122 = Unbundle By Name(w340) -> ("Port"=w339:string, "ConvBox Address"=w338:string, "Assert Ren with IFC"=w337:bool, "System controller"=w336:bool, "IST bit sense"=w335:bool, "GPIB Address"=w334:string)
                n123 = local write "Assert REN w/ IFC"(w337) -> ()
                n124 = local write "ConvBox Port"(w339) -> ()
                n125 = local write "ConvBox Address"(w338) -> ()
                n126 = local write "System Controller"(w336) -> ()
                n127 = local write "IST Bit Sense"(w335) -> ()
                n128 = local write "GPIB Address"(w334) -> ()
              }
            }
            n129 = To Unsigned Long Integer(number=w271) -> (unsigned 32bit integer=w274:u32)
            n130 = local write "Protocol Settings"(w274) -> ()
            n131 = local write "Protocol"(w273) -> ()
            n132 = case shown="False" w266 {
              tunnel: w270 -> [w285 _]
              tunnel: w269 -> [w284 _]
              tunnel: w268 -> [w283 w286]
              tunnel: [w282 w286] -> w267
              frame False {
                n133 = call "Set Codes on all Error Channels.vi"("error in (no error)"=w283, "Error Codes"=w285, "Node Ptr in"=w284) -> ("error out"=w282:errorcluster)  [unwired: 7 in, 1 out]
              }
              frame True {
              }
            }
          }
        }
        n134 = call <vilib>:"Simple Error Handler.vi"("error in (no error)"=w56) -> ("error out"=w55:errorcluster)  [unwired: 1 in, 7 out]
        n135 = call <vilib>:"Clear Errors.vi"("error in (no error)"=w55) -> ("error out"=w54:errorcluster)  [unwired: 1 in, 5 out]
      }
      n136 = Unregister For Events(event registration refnum=w47, error in=w46) -> (error out=w45:errorcluster)
    }
    frame Error {
      n137 = call <vilib>:"Simple Error Handler.vi"("error in (no error)"=w347) -> ("error out"=w346:errorcluster)  [unwired: 1 in, 7 out]
      n138 = call <vilib>:"Clear Errors.vi"("error in (no error)"=w346) -> ("error out"=w345:errorcluster)  [unwired: 1 in, 5 out]
    }
  }
  n139 = invoke class="VI" method="FP.Close"(error in=w12) -> (error out=w11:errorcluster)  [unwired: 2 in, 2 out]
  n140 = call <vilib>:"NI VeriStand - Signal When Ready for Shutdown.vi"("error in (no error)"=w11) -> ("error out"=→"error out":errorcluster)  [unwired: 10 out]
